vi "Convert_Time_Parameter.vi"(0 "Data":T1 {"Register_Address" format="%x"; "Target_Address" format="%x"}) -> (4 "Converted_Data":T2)   [LabVIEW 2023]
uses:
  Controls/Time_Parameter.ctl
  Controls/Converted_Data.ctl
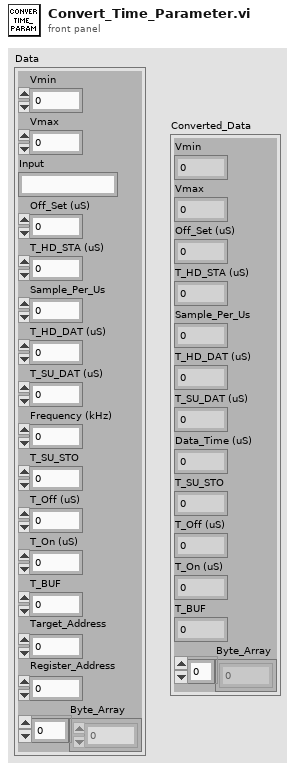
[diagram p1: front panel]
types:
  T1 = typedef "Converted_Data.ctl" = cluster{"Vmin":dbl, "Vmax":dbl, "Input":string, "Off_Set (uS)":dbl, "T_HD_STA (uS)":dbl, "Sample_Per_Us":dbl, "T_HD_DAT (uS)":dbl, "T_SU_DAT (uS)":dbl, "Frequency (kHz)":dbl, "T_SU_STO":dbl, "T_Off (uS)":dbl, "T_On (uS)":dbl, "T_BUF":dbl, "Target_Address":u8, "Register_Address":u8, "Byte_Array":u8[]}
  T2 = typedef "Time_Parameter.ctl" = cluster{"Vmin":dbl, "Vmax":dbl, "Off_Set (uS)":i32, "T_HD_STA (uS)":i32, "Sample_Per_Us":i32, "T_HD_DAT (uS)":i32, "T_SU_DAT (uS)":i32, "Data_Time (uS)":i32, "T_SU_STO":i32, "T_Off (uS)":i32, "T_On (uS)":i32, "T_BUF":i32, "Byte_Array":u8[]}
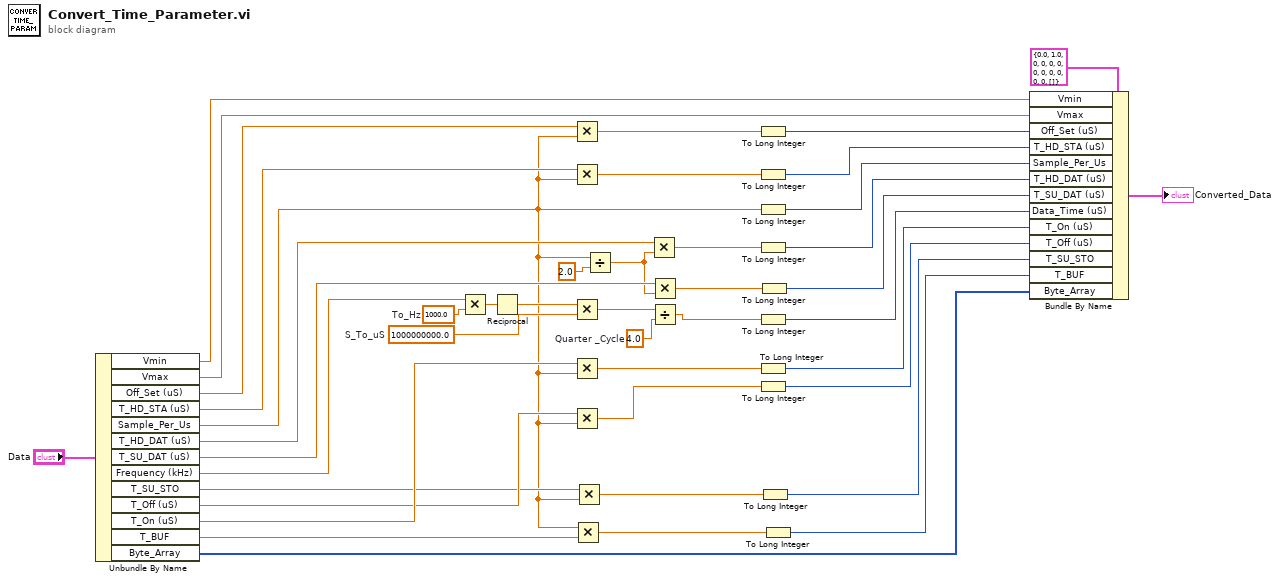
[diagram p0: block diagram]
diagram:
  w12 = 4.0  # Quarter _Cycle
  w8 = 1000.0  # To_Hz
  w14 = 1000000000.0  # S_To_uS
  n1 = Unbundle By Name("Data") -> ("Vmin"=w31:dbl, "Vmax"=w32:dbl, "Off_Set (uS)"=w26:dbl, "T_HD_STA (uS)"=w25:dbl, "Sample_Per_Us"=w4:dbl, "T_HD_DAT (uS)"=w24:dbl, "T_SU_DAT (uS)"=w23:dbl, "Frequency (kHz)"=w22:dbl, "T_SU_STO"=w19:dbl, "T_Off (uS)"=w20:dbl, "T_On (uS)"=w21:dbl, "T_BUF"=w3:dbl, "Byte_Array"=w1:u8[])
  n2 = Multiply(x=w22, y=w8) -> (x*y=w7:dbl)
  n3 = Reciprocal(x=w7) -> (1/x=w6:dbl)
  n4 = Multiply(x=w26, y=w4) -> (x*y=w9:dbl)
  n5 = Multiply(x=w25, y=w4) -> (x*y=w10:dbl)
  n6 = Multiply(x=w6, y=w14) -> (x*y=w11:dbl)
  n7 = Multiply(x=w21, y=w4) -> (x*y=w29:dbl)
  n8 = Multiply(x=w20, y=w4) -> (x*y=w28:dbl)
  n9 = Multiply(x=w4, y=w3) -> (x*y=w2:dbl)
  n10 = Multiply(x=w19, y=w4) -> (x*y=w15:dbl)
  n11 = Divide(x=w4, y=2.0) -> (x/y=w17:dbl)
  n12 = Multiply(x=w24, y=w17) -> (x*y=w27:dbl)
  n13 = Multiply(x=w23, y=w17) -> (x*y=w13:dbl)
  n14 = Divide(x=w11, y=w12) -> (x/y=w5:dbl)
  n15 = To Long Integer(number=w9) -> (32bit integer=w33:i32)
  n16 = To Long Integer(number=w10) -> (32bit integer=w34:i32)
  n17 = To Long Integer(number=w4) -> (32bit integer=w35:i32)
  n18 = To Long Integer(number=w27) -> (32bit integer=w36:i32)
  n19 = To Long Integer(number=w5) -> (32bit integer=w38:i32)
  n20 = To Long Integer(number=w29) -> (32bit integer=w39:i32)
  n21 = To Long Integer(number=w28) -> (32bit integer=w40:i32)
  n22 = To Long Integer(number=w13) -> (32bit integer=w37:i32)
  n23 = To Long Integer(number=w15) -> (32bit integer=w41:i32)
  n24 = To Long Integer(number=w2) -> (32bit integer=w42:i32)
  n25 = Bundle By Name(cluster=T2 {"Vmin"=0.0, "Vmax"=1.0, "Off_Set (uS)"=0, "T_HD_STA (uS)"=0, "Sample_Per_Us"=0, "T_HD_DAT (uS)"=0, "T_SU_DAT (uS)"=0, "Data_Time (uS)"=0, "T_SU_STO"=0, "T_Off (uS)"=0, "T_On (uS)"=0, "T_BUF"=0, "Byte_Array"=[]}, "Vmin"=w31, "Vmax"=w32, "Off_Set (uS)"=w33, "T_HD_STA (uS)"=w34, "Sample_Per_Us"=w35, "T_HD_DAT (uS)"=w36, "T_SU_DAT (uS)"=w37, "Data_Time (uS)"=w38, "T_On (uS)"=w39, "T_Off (uS)"=w40, "T_SU_STO"=w41, "T_BUF"=w42, "Byte_Array"=w1) -> (→"Converted_Data":T2)
